vi "V4.2校准列表.vi"(7 "功能":enum16{"读取", "写入"}(ring), 8 "error in (no error)":errorcluster caption="错误输入（无错误）", 10 "校准参数 in":T1 {"拟合方法" items=["线性", "多项式", "折线"]}, 11 "MB session in":refnum<class "MB_Master.lvclass">) -> (0 "error out":errorcluster caption="错误输出", 2 "校准参数 out":T1 {"拟合方法" items=["线性", "多项式", "折线"]}, 3 "MB session out":refnum<class "MB_Master.lvclass">)   [LabVIEW 2016, in "斯坦道氟化物.lvlib"]
uses:
  <vilib>/Plasmionique/MB Master/MB_Master/MB_Master.lvclass
  <vilib>/Plasmionique/MB Master/MB Master.lvlib
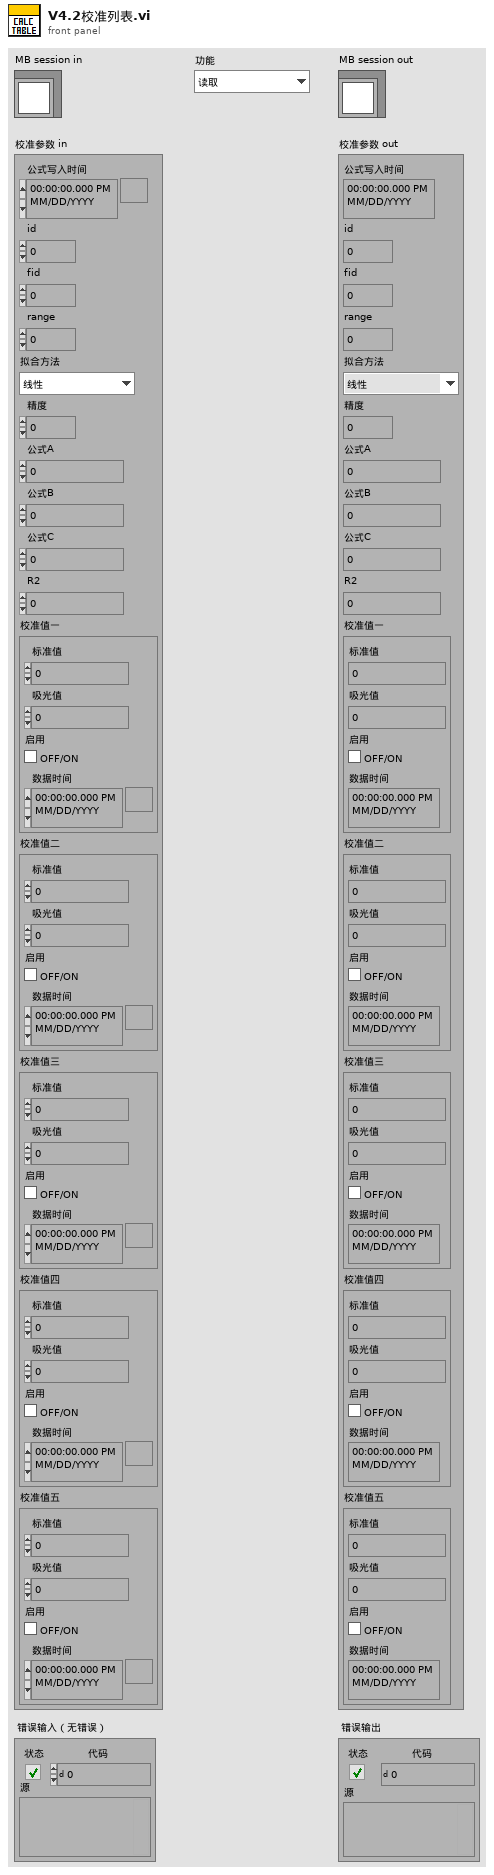
[diagram p1: front panel]
types:
  T1 = typedef "斯坦道氟化物.lvlib/校准参数.ctl" = cluster{"公式写入时间":timestamp, "id":u8, "fid":u8, "range":u8, "拟合方法":u16, "精度":u16, "公式A":sgl, "公式B":sgl, "公式C":sgl, "R2":sgl, "校准值一":cluster{"标准值":sgl, "吸光值":sgl, "启用":bool, "数据时间":timestamp}, "校准值二":cluster{"标准值":sgl, "吸光值":sgl, "启用":bool, "数据时间":timestamp}, "校准值三":cluster{"标准值":sgl, "吸光值":sgl, "启用":bool, "数据时间":timestamp}, "校准值四":cluster{"标准值":sgl, "吸光值":sgl, "启用":bool, "数据时间":timestamp}, "校准值五":cluster{"标准值":sgl, "吸光值":sgl, "启用":bool, "数据时间":timestamp}}
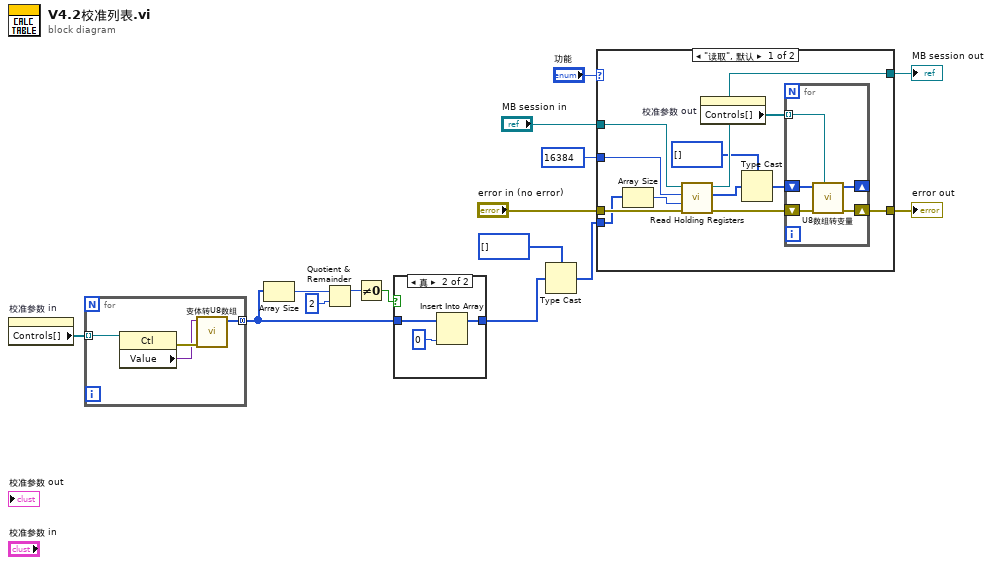
[diagram p0: block diagram]
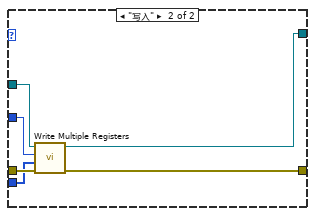
[diagram p2: hidden frame]
diagram:
  n1 = property on="校准参数 in" class="Clust (严格)"() -> ("Controls[]"=w15:refnum<vi>[])  [unwired: 2 in, 2 out]
  n2 = for {
    tunnel: w15 -> [w19] mode=indexing
    tunnel: [w17] -> w10 mode=concatenating
    n3 = property class="Ctl"(reference=w19) -> (error out=w18:errorcluster, "Value"=w16:variant)  [unwired: 1 in, 1 out]
    n4 = call "变体转U8数组.vi"("错误输入（无错误）"=w18, "Value"=w16) -> ("U8数组"=w17:u8[])  [unwired: 8 in, 1 out]
  }
  n5 = Array Size(array=w10) -> (size(s)=w13:i32)
  n6 = Quotient & Remainder(x=w13, y=2) -> (x-y*floor(x/y)=w12:i32)  [unwired: 1 out]
  n7 = Not Equal To 0?(x=w12) -> (x != 0?=w11:bool)
  n8 = case shown="真" w11 {
    tunnel: w10 -> [w20 w23]
    tunnel: [w20 w21] -> w2
    frame False {
    }
    frame True {
      n9 = Insert Into Array(array=w23, new element=u8 0 ("新元素/子数组")) -> (w21:u8[])  [unwired: 1 in]
    }
  }
  n10 = Type Cast(type=u16[] [], x=w2) -> (*(type *) &x=w1:u16[])
  n11 = case shown="\"读取\", 默认" "功能" {
    tunnel: "error in (no error)" -> [w33 w46]
    tunnel: [w29 w45] -> w8
    tunnel: [w34 w44] -> w7
    tunnel: "MB session in" -> [w35 w43]
    tunnel: u16 16384 ("starting address") -> [w32 w42]
    tunnel: w1 -> [w25 w41]
    frame "读取", Default {
      n12 = Array Size(array=w25) -> (size(s)=w24:i32)
      n13 = call <vilib>:"Read Holding Registers.vi"("error in (no error)"=w33, "quantity"=w24, "starting address"=w32, "MB session in"=w35) -> ("error out"=w30:errorcluster, "Registers"=w27:u16[], "MB session out"=w34:refnum<class "MB_Master.lvclass">)  [unwired: 5 in]
      n14 = property on="校准参数 out" class="Clust (严格)"() -> ("Controls[]"=w31:refnum<vi>[])  [unwired: 2 in, 2 out]
      n15 = Type Cast(type=u8[] [], x=w27) -> (*(type *) &x=w26:u8[])
      n16 = for {
        shift-right: [w39] -> w29
        shift-left: w30 -> [w40]
        tunnel: w31 -> [w36] mode=indexing
        shift-right: [w38] -> _
        shift-left: w26 -> [w37]
        n17 = call "U8数组转变量.vi"("Control输入"=w36, "错误输入（无错误）"=w40, "数组输入"=w37) -> ("错误输出"=w39:errorcluster, "数组输出"=w38:u8[])  [unwired: 7 in]
      }
    }
    frame "写入" {
      n18 = call <vilib>:"Write Multiple Registers.vi"("error in (no error)"=w46, "values"=w41, "starting address"=w42, "MB session in"=w43) -> ("error out"=w45:errorcluster, "MB session out"=w44:refnum<class "MB_Master.lvclass">)  [unwired: 6 in]
    }
  }
  "error out" <- w8
  "MB session out" <- w7
